vi "Compute FK.vi"(8 "error in (no error)":errorcluster, 11 "joints":dbl[](array[numeric])=[0.0, 0.0, 0.0, 0.0, 0.0, 0.0]) -> (0 "error out":errorcluster, 3 "transform":T1)   [LabVIEW 2013, in "ikfast_labview.lvlib"]
doc: "IKFAST_API void ComputeFk(const IkReal* joints, IkReal* eetrans, IkReal* eerot);"
uses:
  ikfast_labview.lvlib
  <vilib>/Analysis/Matrix/Datatypes/RealMatrix.ctl
  ikfast_labview.dll
  <vilib>/robotics/Kinematics/NI_Kinematics.lvlib
  <vilib>/Analysis/Matrix/NI_Matrix.lvlib
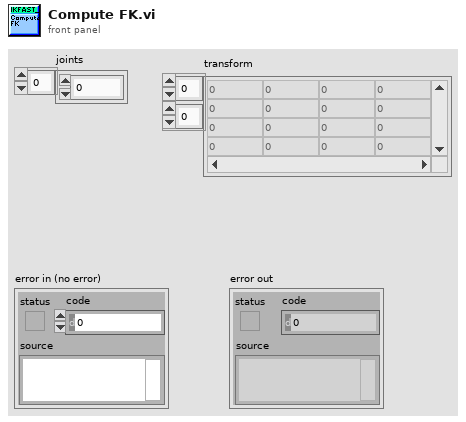
[diagram p1: front panel]
types:
  T1 = typedef "NI_Matrix.lvlib/RealMatrix.ctl" = dbl[][]
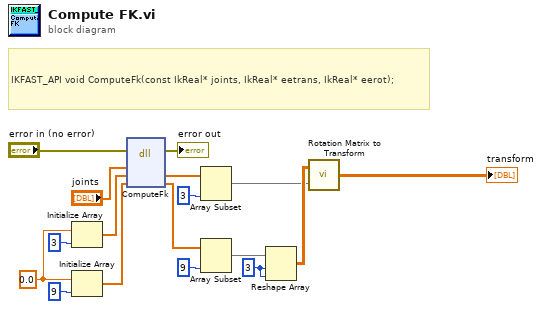
[diagram p0: block diagram]
diagram:
  w9 = 3 ("dimension size")
  w12 = 0.0 ("element")
  # "IKFAST_API void ComputeFk(const IkReal* joints, IkReal* eetrans, IkReal* eerot);"
  n1 = Initialize Array(w12, 3 ("dimension size")) -> (w11:dbl[])
  n2 = Initialize Array(w12, 9 ("dimension size")) -> (w10:dbl[])
  n3 = dll-call lib="C:/Users/fsuarez/git/ikfast_labview/user.lib/ikfast_labview/ikfast_labview.*" fn="ComputeFk"(error in="error in (no error)", "joints"="joints", "translation"=w11, "rotation"=w10) -> (error out=→"error out":errorcluster, "translation"=w2:dbl[], "rotation"=w1:dbl[])  [unwired: 4 in, 1 out]
  n4 = Array Subset(array=w2, length=3) -> (w3:dbl[])  [unwired: 1 in]
  n5 = Array Subset(array=w1, length=9) -> (w5:dbl[])  [unwired: 1 in]
  n6 = Reshape Array(w5, w9, w9) -> (w8:dbl[][])
  n7 = call <vilib>:"Rotation Matrix to Transform.vi"("translation vector"=w3, "rotation matrix"=w8) -> ("transform"=→"transform":T1)
